vi "Write Key String.vi"(6 "Insert If Not Exist(T)":bool=TRUE, 7 "Section Name":string, 8 "error in (no error)":errorcluster, 9 "Key Value":string, 10 "Key Name":string, 11 "Config Data":T1(array[cluster])) -> (0 "error out":errorcluster, 3 "Config Data dup":T1(array[cluster]))   [LabVIEW 2020, in "GUCalibration2.lvlib"]
uses:
  GUCalibration2.lvlib
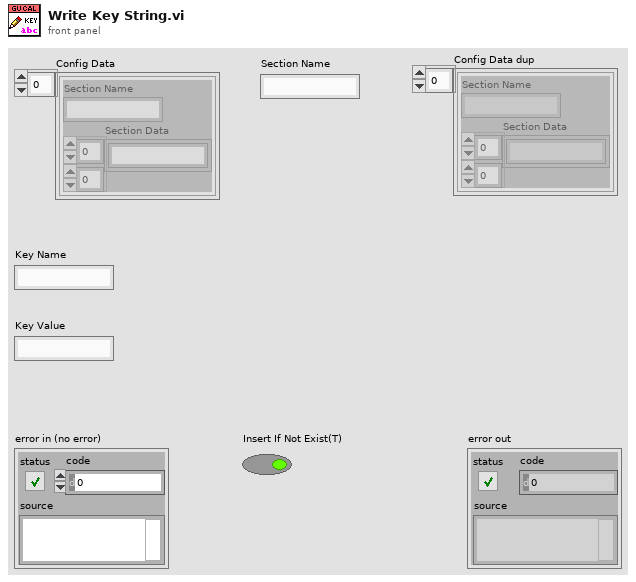
[diagram p1: front panel]
types:
  T1 = cluster{"Section Name":string, "Section Data":string[][]}[]
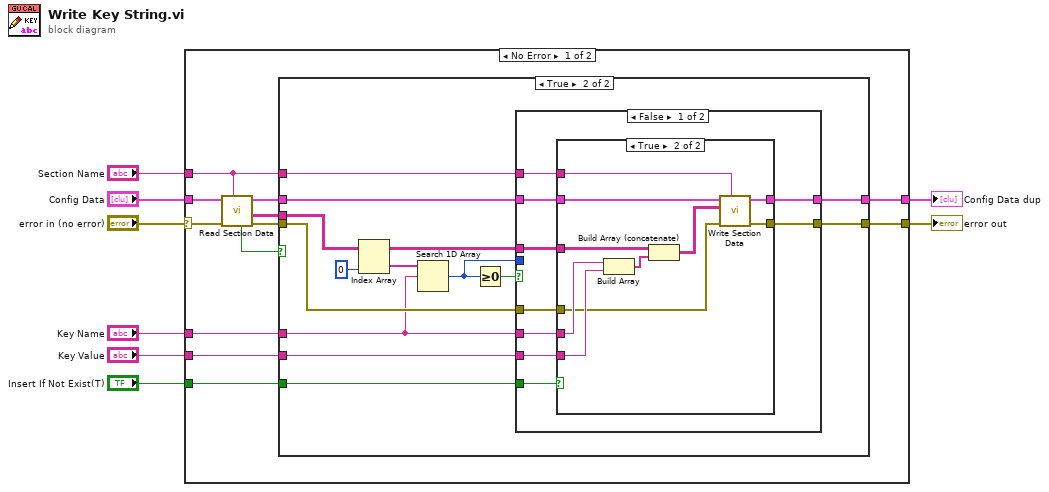
[diagram p0: block diagram]
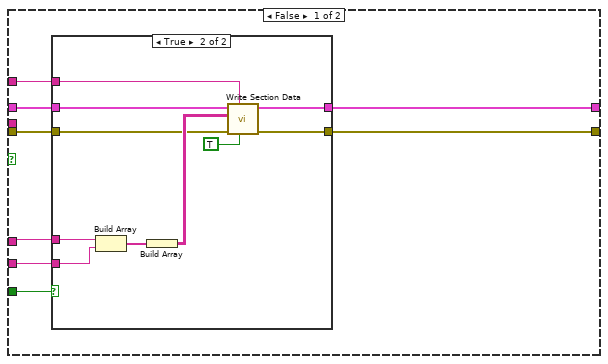
[diagram p2: hidden frame]
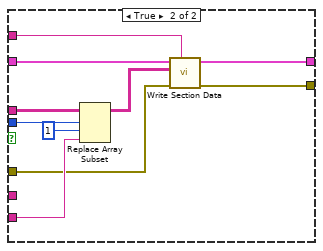
[diagram p5: hidden frame]
diagram:
  n1 = case shown="No Error" "error in (no error)" {
    selector: "error in (no error)" -> [w18 w86]
    tunnel: "Section Name" -> [w10 _]
    tunnel: "Config Data" -> [w19 w85]
    tunnel: [w11 w86] -> w5
    tunnel: [w9 w85] -> w4
    tunnel: "Key Name" -> [w14 _]
    tunnel: "Key Value" -> [w13 _]
    tunnel: "Insert If Not Exist(T)" -> [w12 _]
    frame No Error {
      n2 = call "Read Section Data.vi"("Section Name"=w10, "error in (no error)"=w18, "Config Data"=w19) -> ("error out"=w16:errorcluster, "Section Data"=w20:string[][], "Config Data out"=w15:T1, "Section Exist"=w17:bool)  [unwired: 4 in, 1 out]
      n3 = case shown="True" w17 {
        tunnel: w20 -> [_ w47]
        tunnel: w16 -> [w24 w49]
        tunnel: w15 -> [w27 w50]
        tunnel: w14 -> [w26 w44]
        tunnel: w13 -> [w25 w48]
        tunnel: w12 -> [w21 w45]
        tunnel: [w22 w43] -> w11
        tunnel: w10 -> [w28 w42]
        tunnel: [w23 w41] -> w9
        frame False {
          n4 = case shown="True" w21 {
            tunnel: w28 -> [_ w40]
            tunnel: w27 -> [w30 w39]
            tunnel: w26 -> [_ w38]
            tunnel: w25 -> [_ w37]
            tunnel: w24 -> [w29 w34]
            tunnel: [w30 w32] -> w23
            tunnel: [w29 w31] -> w22
            frame False {
            }
            frame True {
              n5 = Build Array(w38, w37) -> (w36:string[])
              n6 = Build Array(w36) -> (w35:string[][])
              n7 = call "Write Section Data.vi"("Insert If Not Exist(T)"=TRUE, "Section Name"=w40, "error in (no error)"=w34, "Section Data"=w35, "Config Data"=w39) -> ("error out"=w31:errorcluster, "Config Data out"=w32:T1)  [unwired: 5 in]
            }
          }
        }
        frame True {
          n8 = Index Array(array=w47, index (col)=0 ("disabled index (col)")) -> (element=w53:string[])  [unwired: 1 in]
          n9 = Search 1D Array(1D array=w53, element=w44) -> (index of element=w46:i32)  [unwired: 1 in]
          n10 = Greater Or Equal To 0?(x=w46) -> (x >= 0?=w51:bool)
          n11 = case shown="False" w51 {
            tunnel: w50 -> [w56 w78]
            tunnel: w49 -> [w61 w80]
            tunnel: w48 -> [w59 w83]
            tunnel: w47 -> [w58 w84]
            tunnel: w46 -> [_ w82]
            tunnel: w45 -> [w62 _]
            tunnel: w44 -> [w60 _]
            tunnel: [w57 w75] -> w43
            tunnel: w42 -> [w54 w77]
            tunnel: [w55 w76] -> w41
            frame False {
              n12 = case shown="True" w62 {
                tunnel: w61 -> [w64 w70]
                tunnel: w60 -> [_ w74]
                tunnel: w59 -> [_ w73]
                tunnel: w58 -> [_ w72]
                tunnel: [w64 w69] -> w57
                tunnel: w56 -> [w63 w68]
                tunnel: [w63 w67] -> w55
                tunnel: w54 -> [_ w66]
                frame False {
                }
                frame True {
                  n13 = Build Array(w74, w73) -> (w71:string[])
                  n14 = Build Array (concatenate)(w72, w71) -> (w65:string[][])
                  n15 = call "Write Section Data.vi"("Section Name"=w66, "error in (no error)"=w70, "Section Data"=w65, "Config Data"=w68) -> ("error out"=w69:errorcluster, "Config Data out"=w67:T1)  [unwired: 6 in]
                }
              }
            }
            frame True {
              n16 = Replace Array Subset(array=w84, new element=w83, index (row)=w82, index (col)=1 ("disabled index (col)")) -> (w79:string[][])
              n17 = call "Write Section Data.vi"("Section Name"=w77, "error in (no error)"=w80, "Section Data"=w79, "Config Data"=w78) -> ("error out"=w75:errorcluster, "Config Data out"=w76:T1)  [unwired: 6 in]
            }
          }
        }
      }
    }
    frame Error {
    }
  }
  "error out" <- w5
  "Config Data dup" <- w4
